vi "Get Setpoint.vi"(8 "error in":errorcluster, 10 "Ident":string, 11 "Task Actor in":refnum<class "Task Actor.lvclass">) -> (0 "error out":errorcluster, 1 "Data":variant, 3 "Task Actor out":refnum<class "Task Actor.lvclass">)   [LabVIEW 2024, in "Task Actor.lvlib" / "Task Actor.lvclass"]
uses:
  Task Actor.lvclass
  Task Actor.lvclass/Task Actor.ctl
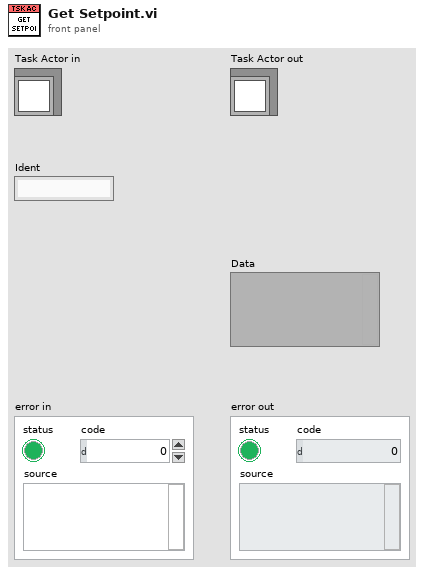
[diagram p1: front panel]
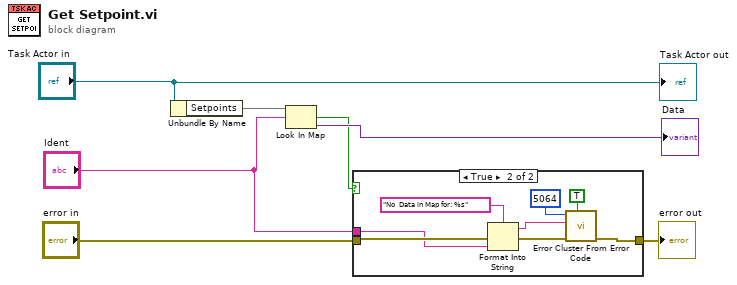
[diagram p0: block diagram]
diagram:
  n1 = Unbundle By Name("Task Actor in") -> ("Setpoints"=w6:map{string, variant})
  n2 = Look In Map(map=w6, key="Ident") -> (key not found?=w3:bool, value=→"Data":variant)  [unwired: 1 in]
  n3 = case shown="True" w3 {
    tunnel: "error in" -> [w8 w14]
    tunnel: "Ident" -> [_ w12]
    tunnel: [w8 w9] -> w1
    frame False {
    }
    frame True {
      n4 = Format Into String(format string="No  Data in Map for: %s" ("error message (\"\")"), error in=w14, w12) -> (resulting string=w11:string, error out=w13:errorcluster)  [unwired: 1 in]
      n5 = call <vilib>:"Error Cluster From Error Code.vi"("show call chain? (False)"=TRUE, "error in (no error)"=w13, "error message (\"\")"=w11, "error code (0)"=5064) -> ("error out"=w9:errorcluster)  [unwired: 5 in]
    }
  }
  "error out" <- w1
  "Task Actor out" <- "Task Actor in"
